vi "수동SubVi.vi"(8 "숫자형 4":dbl, 9 "숫자형 3":dbl, 10 "숫자형":dbl, 11 "숫자형 2":dbl) -> (1 "숫자형 5":dbl)   [LabVIEW 2020]
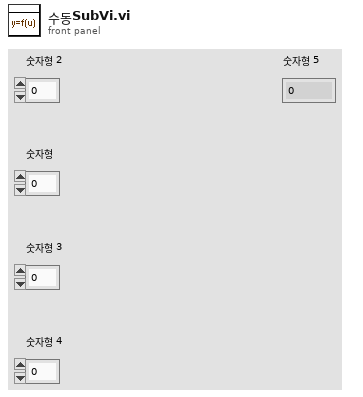
[diagram p1: front panel]
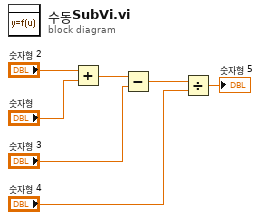
[diagram p0: block diagram]
diagram:
  n1 = Add(x="숫자형 2", y="숫자형") -> (x+y=w3:dbl)
  n2 = Subtract(x=w3, y="숫자형 3") -> (x-y=w1:dbl)
  n3 = Divide(x=w1, y="숫자형 4") -> (x/y=→"숫자형 5":dbl)
